vi "color_loop.vi"() -> ()   [LabVIEW 2014]
panel:
  in  "Stop Button":bool
  in  "milliseconds to wait":u32
  out "Color":u32(colorbox)
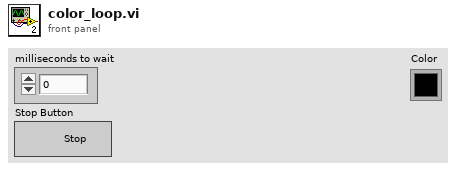
[diagram p1: front panel]
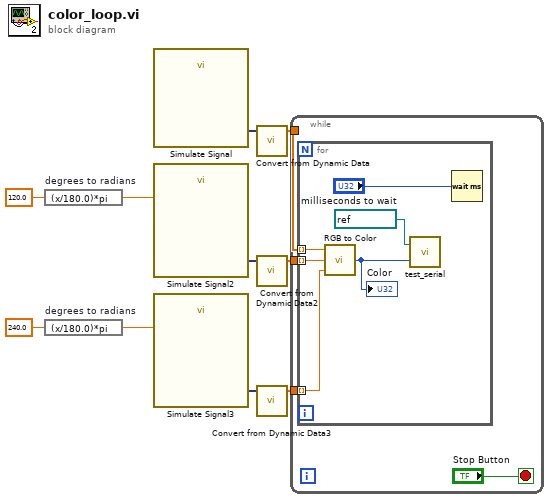
[diagram p0: block diagram]
diagram:
  n1 = expression code="(x/180.0)*pi" "degrees to radians"(120.0) -> (w8:dbl)
  n2 = expression code="(x/180.0)*pi" "degrees to radians"(240.0) -> (w7:dbl)
  n3 = call "Simulate Signal"() -> ("Sine"=w6:dynamicdata)  [unwired: 14 in, 1 out]
  n4 = call "Simulate Signal2"("Phase"=w8) -> ("Sine"=w5:dynamicdata)  [unwired: 13 in, 1 out]
  n5 = call "Simulate Signal3"("Phase"=w7) -> ("Sine"=w4:dynamicdata)  [unwired: 13 in, 1 out]
  n6 = call "Convert from Dynamic Data"("Dynamic Data Type"=w6) -> ("Array"=w3:dbl[])  [unwired: 3 in]
  n7 = call "Convert from Dynamic Data2"("Dynamic Data Type"=w5) -> ("Array"=w2:dbl[])  [unwired: 3 in]
  n8 = call "Convert from Dynamic Data3"("Dynamic Data Type"=w4) -> ("Array"=w1:dbl[])  [unwired: 3 in]
  n9 = while {
    tunnel: w3 -> [w14]
    tunnel: w2 -> [w13]
    tunnel: w1 -> [w12]
    stop <- "Stop Button" stop-if-true
    n10 = for {
      tunnel: w14 -> [w20] mode=indexing
      tunnel: w13 -> [w19] mode=indexing
      tunnel: w12 -> [w18] mode=indexing
      n11 = call <vilib>:"RGB to Color.vi"("B"=w18, "G"=w19, "R"=w20) -> ("Color"=w15:u32)
      "Color" <- w15
      n12 = call "test_serial.vi"("Color Box"=w15, "VISA resource name"=refnum<visa-resource-name> "COM3") -> ()  [unwired: 1 out]
      n13 = Wait (ms)(milliseconds to wait="milliseconds to wait") -> ()  [unwired: 1 out]
    }
  }
